vi "T_At_Wire_U32.vi"(8 "InitClock(ms)":u32, 11 "U32":u32) -> (0 "Clock(ms)":u32, 3 "U32 Out":u32, 4 "Delta(ms)":u32)   [LabVIEW 2019]
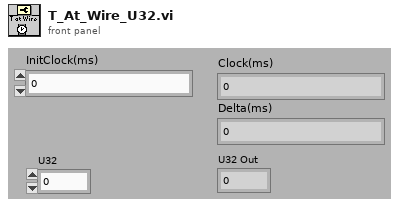
[diagram p1: front panel]
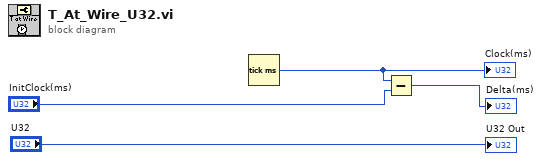
[diagram p0: block diagram]
diagram:
  n1 = Tick Count (ms)() -> (millisecond timer value=w2:u32)
  "Clock(ms)" <- w2
  n2 = Subtract(x=w2, y="InitClock(ms)") -> (x-y=→"Delta(ms)":u32)
  "U32 Out" <- "U32"
